vi "REQ.vi"() -> ()   [LabVIEW 2018]
uses:
  RxTx/RxTx.lvclass
  Channel Req/Channel Req.lvclass
  C:/Users/Denis/Desktop/communication-manager/communication-manager/Communication Channel/Communication Channel.lvclass
  <vilib>/addons/zeromq/zmq_context.lvclass
  Communication Channel/Communication Channel.lvclass
panel:
  in  "Message":string
  in  "Send":bool
  in  "Channel Req.lvclass":refnum<class "Channel Req.lvclass">
  out "error out":errorcluster
  in  "RxTx in":refnum<class "RxTx.lvclass">
  in  "Stop App":bool
  # "REQUEST  example"
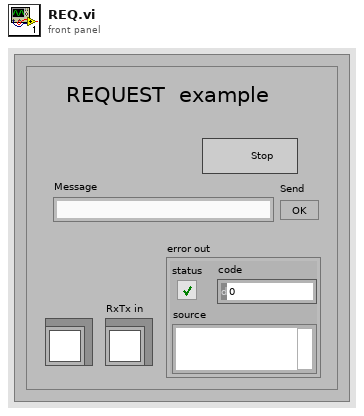
[diagram p1: front panel]
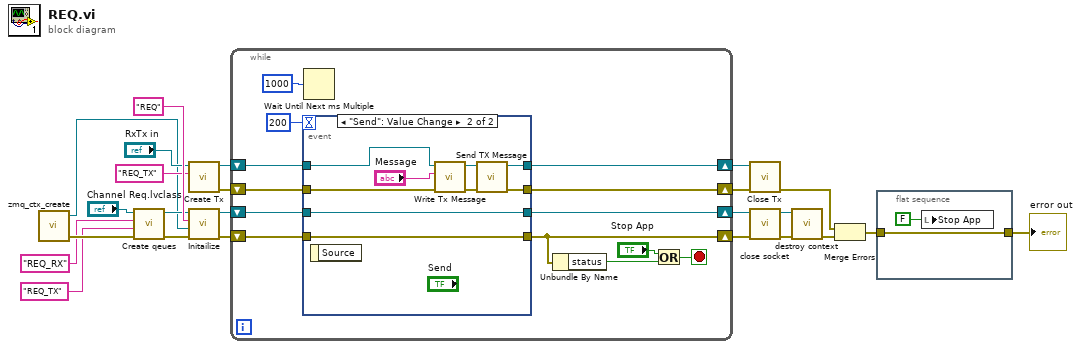
[diagram p0: block diagram]
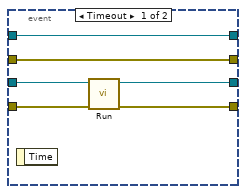
[diagram p2: hidden frame]
diagram:
  n1 = call <vilib>:"zmq_ctx_create.vi"() -> ("error out"=w24:errorcluster, "context out"=w6:refnum<class "zmq_context.lvclass">)  [unwired: 4 in]
  n2 = call "Create qeues.vi"("error in (no error)"=w24, "name qeue Tx"="REQ_TX" ("name qeue Rx"), "name qeue Rx"="REQ_RX", "Communication Channel in"="Channel Req.lvclass") -> ("error out"=w17:errorcluster, "Communication Channel out"=w18:refnum<class "Channel Req.lvclass">)  [unwired: 6 in]
  n3 = call "Create Tx.vi"("Writer Name"="REQ_TX", "RxTx in"="RxTx in") -> ("error out"=w13:errorcluster, "RxTx out"=w14:refnum<class "RxTx.lvclass">)  [unwired: 8 in]
  n4 = call-dynamic "Initailize.vi"("error in (no error)"=w17, "zeromq.lvlib:ZeroMQ Context"=w6, "Name"="REQ", "Channel Req in"=w18) -> ("error out"=w22:errorcluster, "Channel Req out"=w23:refnum<class "Channel Req.lvclass">)  [unwired: 6 in]
  n5 = while {
    shift-right: [w35] -> w20
    shift-left: w23 -> [w37]
    shift-right: [w32] -> w19
    shift-left: w22 -> [w36]
    shift-right: [w34] -> w11
    shift-left: w14 -> [w27]
    shift-right: [w33] -> w10
    shift-left: w13 -> [w28]
    stop <- w29 stop-if-true
    n6 = event shown="[1] \"Send\": Value Change" {
      selector: _ -> [_ _]
      dyn-events: _ -> [_ _]
      timeout: 200 -> [_ _]
      tunnel: w37 -> [w43 w46]
      tunnel: w36 -> [w42 w45]
      tunnel: [w41 w46] -> w35
      tunnel: [w38 w47] -> w34
      tunnel: [w39 w48] -> w33
      tunnel: [w40 w45] -> w32
      tunnel: w28 -> [w39 w49]
      tunnel: w27 -> [w38 w50]
      event Timeout {
        n7 = event-data() -> ()  [unwired: 1 in, 1 out]
        n8 = call-dynamic "Run.vi"("error in (no error)"=w42, "Channel Req in"=w43) -> ("error out"=w40:errorcluster, "Channel Req out"=w41:refnum<class "Channel Req.lvclass">)  [unwired: 8 in]
      }
      event "Send": Value Change {
        n9 = event-data() -> ()  [unwired: 1 in, 1 out]
        n10 = call "Write Tx Message.vi"("error in (no error)"=w49, "Tx Message"="Message", "RxTx in"=w50) -> ("error out"=w51:errorcluster, "RxTx out"=w52:refnum<class "RxTx.lvclass">)  [unwired: 7 in]
        n11 = call "Send TX Message.vi"("error in (no error)"=w51, "RxTx in"=w52) -> ("error out"=w48:errorcluster, "RxTx out"=w47:refnum<class "RxTx.lvclass">)  [unwired: 8 in]
      }
    }
    n12 = Wait Until Next ms Multiple(millisecond multiple=u32 1000) -> ()  [unwired: 1 out]
    n13 = Unbundle By Name(w32) -> ("status"=w31:bool)
    n14 = Or(x="Stop App", y=w31) -> (x .or. y?=w29:bool)
  }
  n15 = call "Close Tx.vi"("error in (no error)"=w10, "RxTx in"=w11) -> ("error out"=w5:errorcluster)  [unwired: 8 in, 1 out]
  n16 = call "close socket.vi"("error in (no error)"=w19, "Communication Channel in"=w20) -> ("error out"=w8:errorcluster, "Communication Channel out"=w7:refnum<class "Channel Req.lvclass">)  [unwired: 8 in]
  n17 = call "destroy context.vi"("error in (no error)"=w8, "Communication Channel in"=w7) -> ("error out"=w4:errorcluster)  [unwired: 8 in, 1 out]
  n18 = Merge Errors(w5, w4) -> (w3:errorcluster)
  n19 = flat-sequence {
    tunnel: w3 -> [w54]
    tunnel: [w54] -> w2
    frame #0 {
      n20 = local write "Stop App"(FALSE ("Stop App")) -> ()
    }
  }
  "error out" <- w2
